vi "read adc.vi"(8 "error in (no error)":errorcluster, 9 "streaming":i32, 10 "handle":u64) -> (0 "error out":errorcluster, 1 "function return":i32, 2 "packet out":T1)   [LabVIEW 2017, in "buddy.lvlib"]
doc: "EXPORT int buddy_read_adc(hid_device *handle, general_packet_t *packet, bool streaming);"
uses:
  buddy.lvlib
  buddy_x64.dll
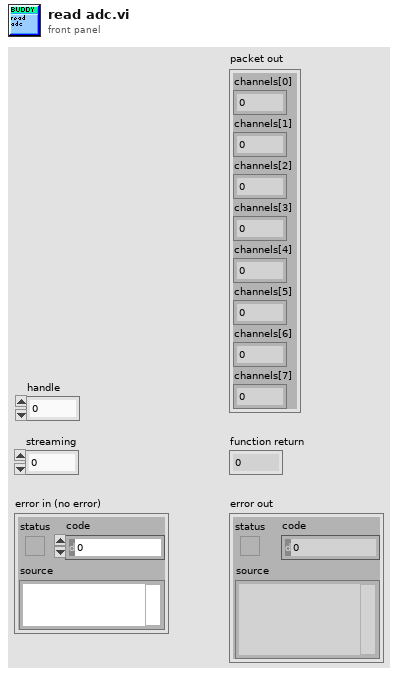
[diagram p1: front panel]
types:
  T1 = cluster{"channels[0]":u16, "channels[1]":u16, "channels[2]":u16, "channels[3]":u16, "channels[4]":u16, "channels[5]":u16, "channels[6]":u16, "channels[7]":u16}
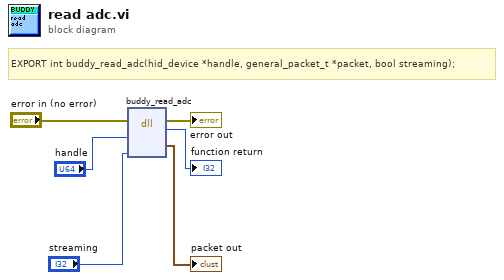
[diagram p0: block diagram]
diagram:
  # "EXPORT int buddy_read_adc(hid_device *handle, general_packet_t *packet, bool streaming);"
  n1 = dll-call lib="C:/Users/shraken/shraken_code/usbhid_buddy/lib/libbuddy/bindings/labview/utility_vi/buddy_x64.dll" fn="buddy_read_adc"(error in="error in (no error)", "handle"="handle", "streaming"="streaming") -> (error out=→"error out":errorcluster, "return type"=→"function return":i32, "packet out"=→"packet out":T1)  [unwired: 5 in, 1 out]
